vi "publishStateChangedEvent.vi"(8 "error in (no error)":errorcluster, 11 "Model in":refnum<class "Model.lvclass">) -> (0 "error out":errorcluster, 3 "Model out":refnum<class "Model.lvclass">)   [LabVIEW 2016, in "Model.lvclass"]
uses:
  Model.lvclass
  Types/StateChangedEvent.ctl
  Types/Timestamp.ctl
  Types/SummaryStates.ctl
  Types/DetailedStates.ctl
  Model.lvclass/Model.ctl
  UserEvents/UserEvents.lvclass/UserEvents.ctl
  Types/M1M3SupportTypes.lvlib
  UserEvents/UserEvents.lvclass
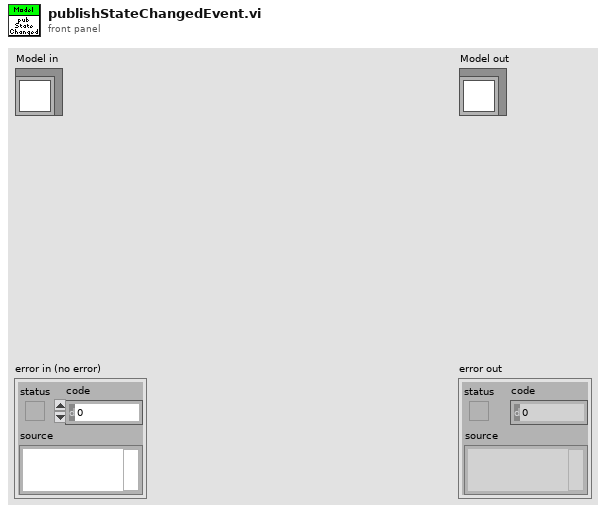
[diagram p1: front panel]
types:
  T1 = typedef "M1M3SupportTypes.lvlib/StateChangedEvent.ctl" = cluster{"Timestamp":T2, "SummaryStates":T3, "DetailedStates":T4}
  T2 = typedef "M1M3SupportTypes.lvlib/Timestamp.ctl" = dbl
  T3 = typedef "M1M3SupportTypes.lvlib/SummaryStates.ctl" = enum16{"OfflineState", "StandbyState", "DisabledState", "EnabledState", "FaultState"}
  T4 = typedef "M1M3SupportTypes.lvlib/DetailedStates.ctl" = enum16{"PublishOnlyState", "AvailableState", "StandbyState", "DisabledState", "EnabledState", "FaultState"}
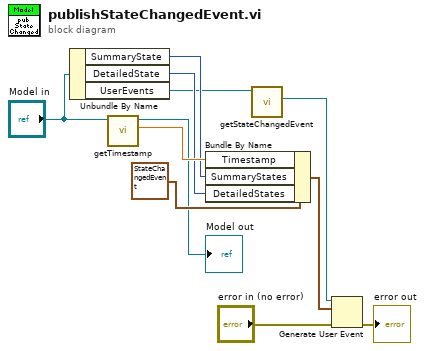
[diagram p0: block diagram]
diagram:
  n1 = Unbundle By Name("Model in") -> ("SummaryState"=w8:T3, "DetailedState"=w7:T4, "UserEvents"=w2:refnum<class "UserEvents.lvclass">)
  n2 = call "getTimestamp.vi"("Model in"="Model in") -> ("Timestamp"=w9:T2, "Model out"=→"Model out":refnum<class "Model.lvclass">)  [unwired: 8 in, 1 out]
  n3 = Bundle By Name(cluster=T1 {"Timestamp"=0.0, "SummaryStates"=enum."OfflineState", "DetailedStates"=enum."PublishOnlyState"} ("event data"), "Timestamp"=w9, "SummaryStates"=w8, "DetailedStates"=w7) -> (w6:T1)
  n4 = call "getStateChangedEvent.vi"("UserEvents in"=w2) -> ("StateChangedEvent"=w1:refnum<user-event>)  [unwired: 9 in, 1 out]
  n5 = Generate User Event(user event=w1, event data cluster=w6, error in="error in (no error)") -> (error out=→"error out":errorcluster)  [unwired: 1 in, 1 out]
